vi "resolve_fast_frames.vi"(3 "fast frame count":i32, 4 "all fast frames":dbl[](array[numeric]), 5 "sample points per frame":i32) -> (1 "resolved waveforms":dbl[][](array[numeric]))   [LabVIEW 2012]
doc: "This vis takes the fast frame waveform measured by the OSC and creates a seperate array for every frame."
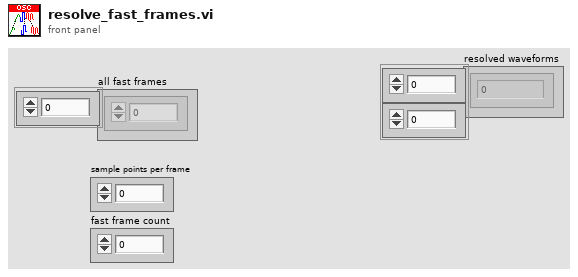
[diagram p1: front panel]
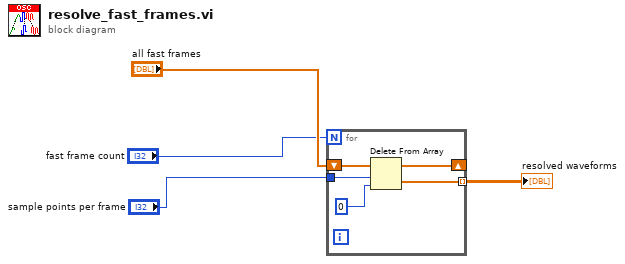
[diagram p0: block diagram]
diagram:
  n1 = for {
    N: "fast frame count" -> [_]
    shift-right: [w8] -> _
    shift-left: "all fast frames" -> [w9]
    tunnel: [w7] -> w2 mode=indexing
    tunnel: "sample points per frame" -> [w6]
    n2 = Delete From Array(array=w9, length=w6, index=u8 0) -> (deleted portion=w7:dbl[], array with subset deleted=w8:dbl[])
  }
  "resolved waveforms" <- w2
